vi "close_i2c_interface.vi"(8 "error in":errorcluster, 10 "I2C interface":T1) -> (0 "error out":errorcluster)   [LabVIEW 2013]
uses:
  i2c_interface.ctl
  fpga_reference.ctl
  <vilib>/Utility/error.llb/Error Cluster From Error Code.vi
  <vilib>/rvi/errors/niLvFpgaAdjustHostInterfaceError.vi
  <vilib>/FPGAPlugInAG/PCIe-7842R/niLvFpga_Close_PCIe-7842R.vi
  <vilib>/rvi/interface/nirviReadWriteControl/nirviReadWriteControl.xnode
  FPGA Bitfiles/i2cmuxdemux.lvbitx
  <vilib>/rvi/interface/nirviCloseFPGA/nirviCloseFPGA.xnode
  NiFpgaLv.dll
panel:
  # "Close I2C FPGA interface, cleaning up resources."
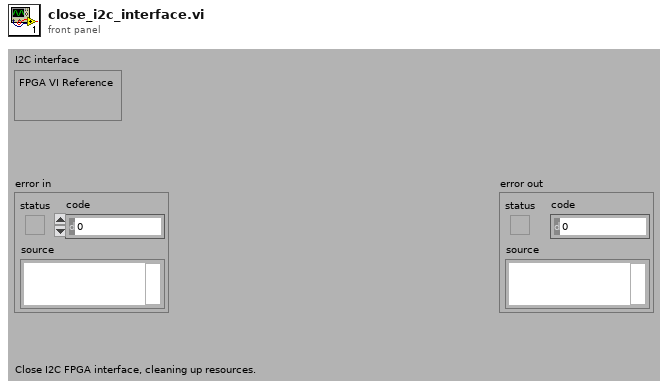
[diagram p1: front panel]
types:
  T1 = typedef "i2c_interface.ctl" = cluster{"FPGA VI Reference":T2}
  T2 = typedef "fpga_reference.ctl" = refnum<k20>
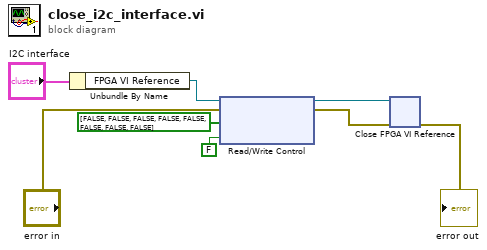
[diagram p0: block diagram]
diagram:
  n1 = Unbundle By Name("I2C interface") -> ("FPGA VI Reference"=w6:T2)
  n2 = xnode "Read/Write Control"("FPGA VI Reference In"=w6, "error in"="error in", "Output enable"=bool[] [FALSE, FALSE, FALSE, FALSE, FALSE, FALSE, FALSE, FALSE], "Finder"=FALSE ("Output Enable")) -> ("FPGA VI Reference Out"=w5:T2, "error out"=w3:errorcluster)
  n3 = xnode "Close FPGA VI Reference"("FPGA VI Reference In"=w5, "error in"=w3) -> ("error out"=→"error out":errorcluster)
